vi "Leds light control.vi"(9 "Control panel":T1, 11 "number":u32) -> (1 "LED 3":bool, 2 "LED 2":bool, 3 "LED 1":bool, 4 "LED 4":bool, 5 "LED 5":bool)   [LabVIEW 2020]
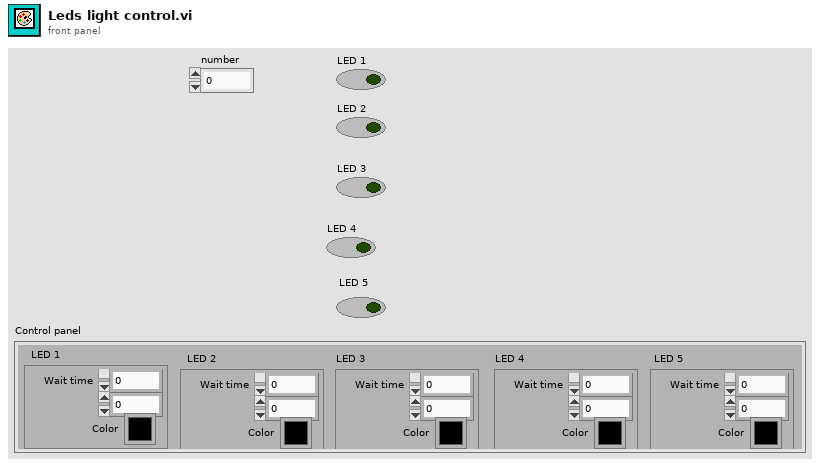
[diagram p1: front panel]
types:
  T1 = cluster{"  LED 1":cluster{"Wait time":dbl, "Duration time":dbl, "Color":u32}, "  LED 2":cluster{"Wait time":dbl, "Duration time":dbl, "Color":u32}, "LED 3":cluster{"Wait time":dbl, "Duration time":dbl, "Color":u32}, "LED 4":cluster{"Wait time":dbl, "Duration time":dbl, "Color":u32}, " LED 5":cluster{"Wait time":dbl, "Duration time":dbl, "Color":u32}}
  T2 = cluster{"Wait time":dbl, "Duration time":dbl, "Color":u32}
  T3 = cluster{"Wait time":dbl, "Wait time":dbl, "Wait time":dbl, "Wait time":dbl, "Wait time":dbl}
  T4 = cluster{"Duration time":dbl, "Duration time":dbl, "Duration time":dbl, "Duration time":dbl, "Duration time":dbl}
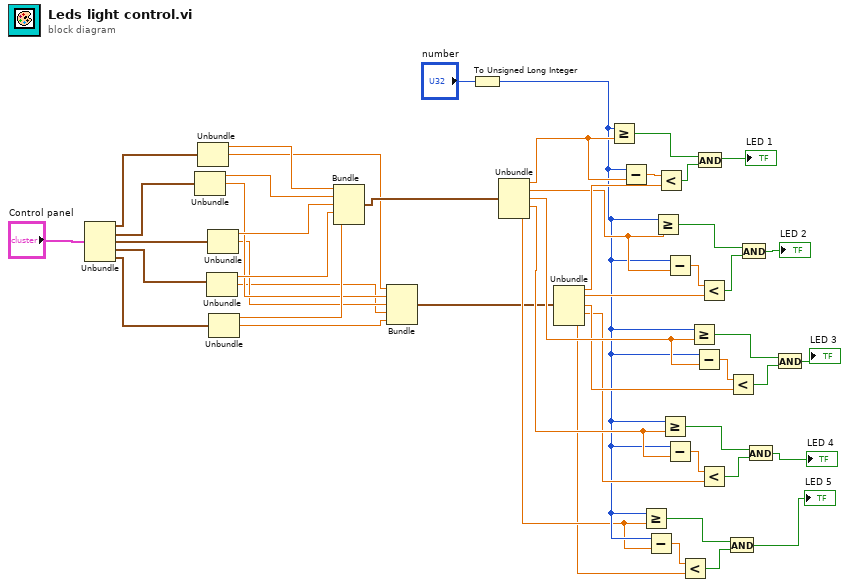
[diagram p0: block diagram]
diagram:
  n1 = Unbundle("Control panel") -> ("LED 1"=w17:T2, "LED 2"=w16:T2, "LED 3"=w15:T2, "LED 4"=w14:T2, "LED 5"=w13:T2)
  n2 = Unbundle(w16) -> ("Wait time"=w11:dbl, "Duration time"=w5:dbl)  [unwired: 1 out]
  n3 = Unbundle(w17) -> ("Wait time"=w12:dbl, "Duration time"=w6:dbl)  [unwired: 1 out]
  n4 = Unbundle(w14) -> ("Wait time"=w9:dbl, "Duration time"=w3:dbl)  [unwired: 1 out]
  n5 = Unbundle(w15) -> ("Wait time"=w10:dbl, "Duration time"=w4:dbl)  [unwired: 1 out]
  n6 = Unbundle(w13) -> ("Wait time"=w8:dbl, "Duration time"=w2:dbl)  [unwired: 1 out]
  n7 = Bundle("Wait time"=w12, "Wait time"=w11, "Wait time"=w10, "Wait time"=w9, "Wait time"=w8) -> (w7:T3)  [unwired: 1 in]
  n8 = Bundle("Duration time"=w6, "Duration time"=w5, "Duration time"=w4, "Duration time"=w3, "Duration time"=w2) -> (w1:T4)  [unwired: 1 in]
  n9 = To Unsigned Long Integer(number="number") -> (unsigned 32bit integer=w21:u32)
  n10 = Unbundle(w7) -> ("Wait time"=w48:dbl, "Wait time"=w40:dbl, "Wait time"=w34:dbl, "Wait time"=w28:dbl, "Wait time"=w20:dbl)
  n11 = Unbundle(w1) -> ("Duration time"=w46:dbl, "Duration time"=w39:dbl, "Duration time"=w33:dbl, "Duration time"=w27:dbl, "Duration time"=w19:dbl)
  n12 = Greater Or Equal?(x=w21, y=w48) -> (x >= y?=w49:bool)
  n13 = Subtract(x=w21, y=w48) -> (x-y=w47:dbl)
  n14 = Greater Or Equal?(x=w21, y=w20) -> (x >= y?=w25:bool)
  n15 = Subtract(x=w21, y=w20) -> (x-y=w24:dbl)
  n16 = Greater Or Equal?(x=w21, y=w40) -> (x >= y?=w43:bool)
  n17 = Less?(x=w47, y=w46) -> (x < y?=w45:bool)
  n18 = Greater Or Equal?(x=w21, y=w28) -> (x >= y?=w31:bool)
  n19 = Subtract(x=w21, y=w40) -> (x-y=w42:dbl)
  n20 = Subtract(x=w21, y=w28) -> (x-y=w30:dbl)
  n21 = Less?(x=w24, y=w19) -> (x < y?=w23:bool)
  n22 = Greater Or Equal?(x=w21, y=w34) -> (x >= y?=w37:bool)
  n23 = Subtract(x=w21, y=w34) -> (x-y=w36:dbl)
  n24 = And(x=w49, y=w45) -> (x .and. y?=→"LED 1":bool)
  n25 = Less?(x=w42, y=w39) -> (x < y?=w41:bool)
  n26 = Less?(x=w30, y=w27) -> (x < y?=w29:bool)
  n27 = And(x=w25, y=w23) -> (x .and. y?=→"LED 5":bool)
  n28 = Less?(x=w36, y=w33) -> (x < y?=w35:bool)
  n29 = And(x=w43, y=w41) -> (x .and. y?=→"LED 2":bool)
  n30 = And(x=w31, y=w29) -> (x .and. y?=→"LED 4":bool)
  n31 = And(x=w37, y=w35) -> (x .and. y?=→"LED 3":bool)
